vi "WorkorderHandler_DefaultData.vi"() -> (0 "data":T1)   [LabVIEW 2011]
doc: "Returns the object data control. You can use this data control as an output from structures and subVIs when an error occurs. Set the values in the data control to the default values for your class object and save as default."
uses:
  DataStructures/WorkorderHandler_ObjectData.ctl
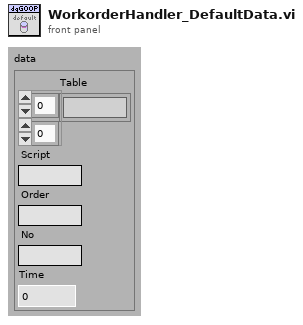
[diagram p1: front panel]
types:
  T1 = typedef "WorkorderHandler_ObjectData.ctl" = cluster{"Table":string[][], "Script":string, "Order":string, "No":string, "Time":dbl}
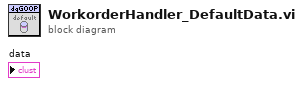
[diagram p0: block diagram]
diagram:
